vi "Event Handler.vi"(8 "error in (no error)":errorcluster, 11 "WebView.JSONEditor in":refnum<class "WebView.JSONEditor.lvclass">) -> ()   [LabVIEW 2024, in "WebView.JSONEditor.lvclass"]
uses:
  WebView.JSONEditor.lvclass
  WebView.JSONEditor.lvclass/WebView.JSONEditor.ctl
  WebView_class/WebView.lvclass
  e3f92d98-e7ad-4bc2-98b6-bd4194dccb6e.vi
  <vilib>/JDP Science/JSONtext/JSONtext.lvlib
  private/JSON Updated Event Data--cluster.ctl
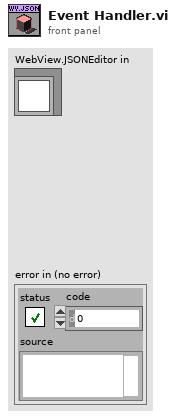
[diagram p1: front panel]
types:
  T1 = typedef "WebView.JSONEditor.lvclass/JSONEditor Events.ctl" = cluster{"JSON Updated":refnum<user-event>, "Selected Node Path":refnum<user-event>}
  T2 = typedef "WebView.lvclass/Events--cluster.ctl" = cluster{"Navigation Complete Event":refnum<user-event>, "Source Changed Event":refnum<user-event>, "Document Title Changed Event":refnum<user-event>, "Status Bar Text Changed":refnum<user-event>, "Web Message Received":refnum<user-event>, "Window Close Requested":refnum<user-event>, "DOM Loaded":refnum<user-event>, "Navigation Started Event":refnum<user-event>}
  T3 = typedef "WebView.JSONEditor.lvclass/JSON Updated Event Data--cluster.ctl" = cluster{"JSON":string}
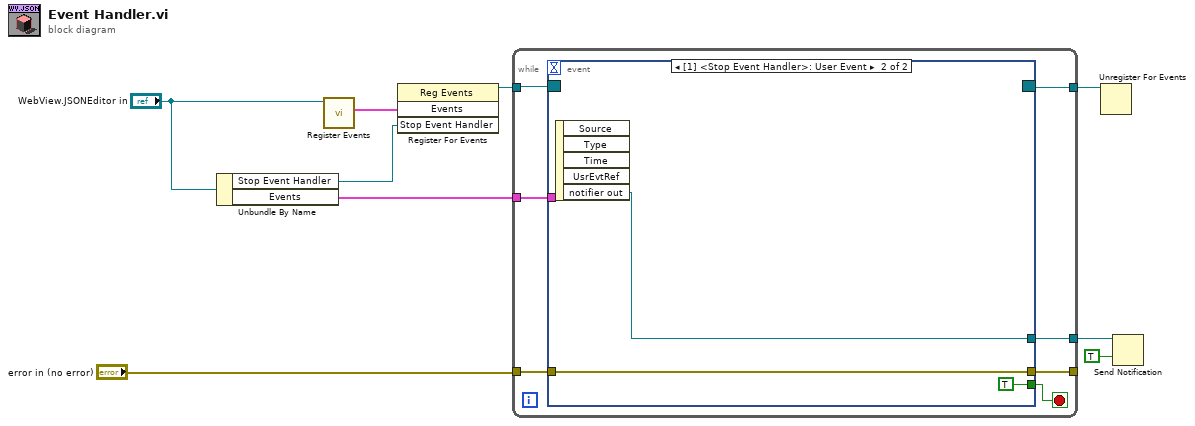
[diagram p0: block diagram]
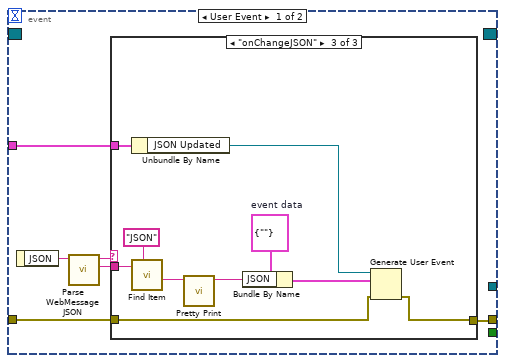
[diagram p2: hidden frame]
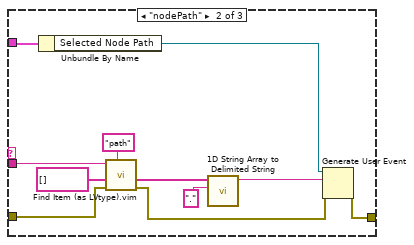
[diagram p4: hidden frame]
diagram:
  n1 = Unbundle By Name("WebView.JSONEditor in") -> ("Stop Event Handler"=w5:refnum<user-event>, "Events"=w3:T1)
  n2 = call-dynamic "Register Events.vi"("WebView in"="WebView.JSONEditor in") -> ("Events"=w7:T2)  [unwired: 8 in, 2 out]
  n3 = register-events(w7, w5) -> (reference out=w8:refnum<event-registration>)  [unwired: 2 in, 1 out]
  n4 = while {
    tunnel: w8 -> [w12]
    tunnel: [w16] -> _
    tunnel: "error in (no error)" -> [w15]
    tunnel: [w13] -> w9
    tunnel: w3 -> [w11]
    tunnel: [w10] -> w2
    stop <- w14 stop-if-true
    n5 = event shown="[1] <Stop Event Handler>: User Event" {
      selector: w12 -> [_ _]
      dyn-events: [_ _] -> w13
      timeout: _ -> [_ _]
      tunnel: [w18 w47] -> w16
      tunnel: w15 -> [w19 w47]
      tunnel: [_ TRUE] -> w14
      tunnel: w11 -> [w17 _]
      tunnel: [_ w45] -> w10
      event User Event {
        n6 = event-data() -> ("JSON"=w22:string)  [unwired: 1 in]
        n7 = call "Parse WebMessage JSON.vi"("JSON in"=w22) -> ("Data out"=w20:string, "Type out"=w21:string)  [unwired: 9 in]
        n8 = case shown="\"onChangeJSON\"" w21 {
          tunnel: w20 -> [_ w34 w40]
          tunnel: w19 -> [w23 w33 w41]
          tunnel: [w23 w27 w42] -> w18
          tunnel: w17 -> [_ w30 w44]
          frame Default {
          }
          frame "nodePath" {
            n9 = Unbundle By Name(w30) -> ("Selected Node Path"=w29:refnum<user-event>)
            n10 = call "Find Item (as LVtype).vim"("$Path or Item Name"="path", "error in (no error)"=w33, "Data Type and Default Value"=string[] [], "JSON"=w34) -> ("error out"=w28:errorcluster, "Data"=w25:string[])  [unwired: 4 in, 2 out]
            n11 = call <vilib>:"1D String Array to Delimited String.vi"("delimiter"=".", "string array"=w25) -> ("delimited string"=w24:string)  [unwired: 9 in]
            n12 = Generate User Event(user event=w29, event data cluster=w24, error in=w28) -> (error out=w27:errorcluster)  [unwired: 1 in, 1 out]
          }
          frame "onChangeJSON" {
            w39 = T3 {"JSON"=""}  # event data
            n13 = Unbundle By Name(w44) -> ("JSON Updated"=w43:refnum<user-event>)
            n14 = call <vilib>:"Find Item.vi"("$Path or Item Name"="JSON", "JSON"=w40) -> ("<JSON>"=w37:string)  [unwired: 6 in, 3 out]
            n15 = call <vilib>:"Pretty Print.vi"("JSON"=w37) -> ("<JSON>"=w35:string)  [unwired: 8 in, 2 out]
            n16 = Bundle By Name(cluster=w39, "JSON"=w35) -> (w38:T3)
            n17 = Generate User Event(user event=w43, event data cluster=w38, error in=w41) -> (error out=w42:errorcluster)  [unwired: 1 in, 1 out]
          }
        }
      }
      event User Event {
        n18 = event-data() -> ("notifier out"=w45:refnum<notifier>)  [unwired: 1 in, 4 out]
      }
    }
  }
  n19 = Unregister For Events(event registration refnum=w9) -> ()  [unwired: 1 in, 1 out]
  n20 = Send Notification(notification=TRUE, notifier=w2) -> ()  [unwired: 1 in, 2 out]
